vi "Path.vi"(1 "selected path":path) -> (8 "Boolean":bool, 9 "appended path":path)   [LabVIEW 2021]
uses:
  <vilib>/Utility/file.llb/Write Delimited Spreadsheet (string).vi
panel:
  out "Exist?":bool
  out "Name":string
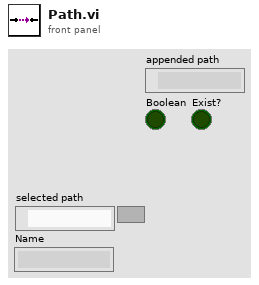
[diagram p1: front panel]
types:
  T1 = enum16{"open", "replace", "create", "open or create", "replace or create", "replace or create with confirmation"}
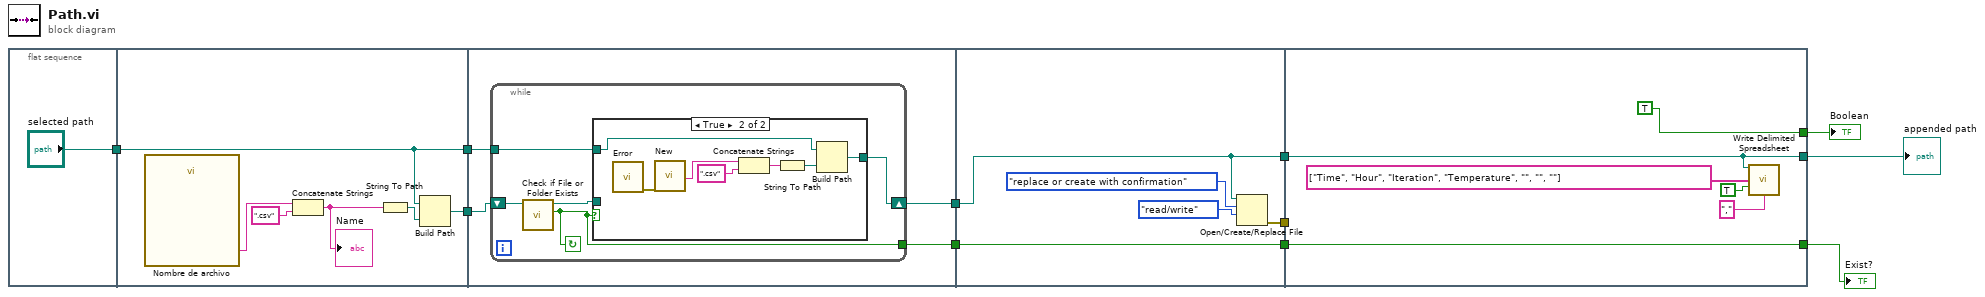
[diagram p0: block diagram]
diagram:
  n1 = flat-sequence {
    tunnel: ["selected path"] -> w11
    tunnel: w11 -> [w13]
    tunnel: [w14] -> w10
    tunnel: [w13] -> w9
    tunnel: w10 -> [w22]
    tunnel: w9 -> [w21]
    tunnel: [w20] -> w8
    tunnel: [w19] -> w7
    tunnel: w8 -> [w39]
    tunnel: w7 -> [w40]
    tunnel: [w39] -> w6
    tunnel: [w40] -> w5
    tunnel: [w36] -> w4
    tunnel: [w46] -> w2
    tunnel: [w45] -> w3
    tunnel: w6 -> [w45]
    tunnel: w5 -> [w46]
    tunnel: w4 -> [_]
    tunnel: [TRUE] -> w1
    frame #0 {
    }
    frame #1 {
      n2 = call "Nombre de archivo"() -> ("Nombre"=w18:string)  [unwired: 17 in, 2 out]
      n3 = Concatenate Strings(w18, ".csv" ("string")) -> (w15:string)
      "Name" <- w15
      n4 = String To Path(string=w15) -> (path=w16:path)
      n5 = Build Path(base path=w13, name or relative path=w16) -> (appended path=w14:path)
    }
    frame #2 {
      n6 = while {
        shift-right: [w25] -> w20
        shift-left: w22 -> [w27]
        tunnel: w21 -> [w26]
        tunnel: [w23] -> w19
        stop <- w23 continue-if-true
        n7 = call <vilib>:"Check if File or Folder Exists.vi"("path"=w27) -> ("file or folder exists?"=w23:bool, "dup path"=w24:path)  [unwired: 8 in, 1 out]
        n8 = case shown="True" w23 {
          tunnel: w26 -> [_ w31]
          tunnel: [w28 w30] -> w25
          tunnel: w24 -> [w28 _]
          frame False {
          }
          frame True {
            n9 = call "Error"() -> ("error out"=w34:errorcluster)  [unwired: 10 in, 1 out]
            n10 = call "New"("error in (no error)"=w34) -> ("Nombre"=w29:string)  [unwired: 16 in, 2 out]
            n11 = Concatenate Strings(w29, ".csv" ("string")) -> (w35:string)
            n12 = String To Path(string=w35) -> (path=w32:path)
            n13 = Build Path(base path=w31, name or relative path=w32) -> (appended path=w30:path)
          }
        }
      }
    }
    frame #3 {
      n14 = Open/Create/Replace File(file path (use dialog)=w39, operation (0:open)=T1."replace or create with confirmation", access (0:read/write)=enum16{"read/write", "read-only", "write-only"}."read/write") -> (error out=w36:errorcluster)  [unwired: 3 in, 2 out]
    }
    frame #4 {
      n15 = call-poly <vilib>:"Write Delimited Spreadsheet.vi"("file path (dialog if empty)"=w45, "1D data"=string[] ["Time", "Hour", "Iteration", "Temperature", "", "", ""] ("row headers"), "append to file? (new file:F)"=TRUE, "delimiter (\\t)"="," ("delimiter (\\t)")) -> ()  [unwired: 10 in, 2 out]
    }
  }
  "appended path" <- w3
  "Boolean" <- w1
  "Exist?" <- w2
